vi "SUB-자료변환-32Bit 데이터를 실수형(float)으로 변환.vi"(3 "U32":u32) -> (1 "FP32":sgl)   [LabVIEW 2015]
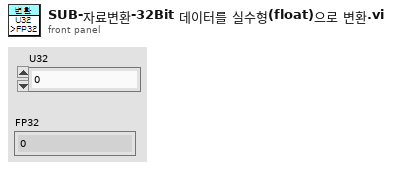
[diagram p1: front panel]
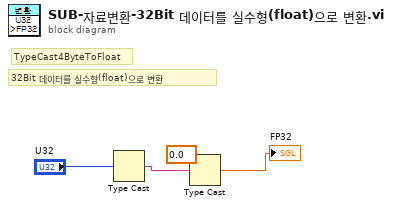
[diagram p0: block diagram]
diagram:
  # "32Bit 데이터를 실수형(float)으로 변환"
  # "TypeCast4ByteToFloat"
  n1 = Type Cast(x="U32") -> (*(type *) &x=w3:string)  [unwired: 1 in]
  n2 = Type Cast(type=sgl 0.0, x=w3) -> (*(type *) &x=→"FP32":sgl)
